vi "Graphics-Get Plot Properties.vi"(0 "Plot in":refnum<vi>, 11 "error in (no error)":errorcluster) -> (4 "Plot out":refnum<vi>, 8 "properties":T1, 15 "error out":errorcluster)   [LabVIEW 2020]
uses:
  Graphics-Plot Properties.ctl
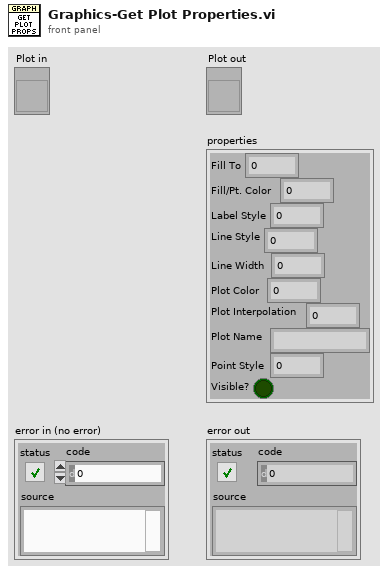
[diagram p1: front panel]
types:
  T1 = typedef "Graphics-Plot Properties.ctl" = cluster{"Fill To":i16, "Fill/Pt. Color":u32, "Label Style":u8, "Line Style":u8, "Line Width":u8, "Plot Color":u32, "Plot Interpolation":u8, "Plot Name":string, "Point Style":u8, "Visible?":bool}
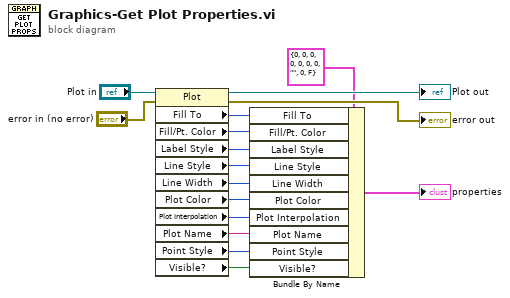
[diagram p0: block diagram]
diagram:
  n1 = property class="Plot"(reference="Plot in", error in="error in (no error)") -> (reference out=→"Plot out":refnum<vi>, error out=→"error out":errorcluster, "Fill To"=w11:i16, "Fill/Pt. Color"=w10:u32, "Label Style"=w9:u8, "Line Style"=w8:u8, "Line Width"=w7:u8, "Plot Color"=w6:u32, "Plot Interpolation"=w5:u8, "Plot Name"=w4:string, "Point Style"=w3:u8, "Visible?"=w2:bool)
  n2 = Bundle By Name(cluster=T1 {"Fill To"=0, "Fill/Pt. Color"=0, "Label Style"=0, "Line Style"=0, "Line Width"=0, "Plot Color"=0, "Plot Interpolation"=0, "Plot Name"="", "Point Style"=0, "Visible?"=FALSE} ("plot properties"), "Fill To"=w11, "Fill/Pt. Color"=w10, "Label Style"=w9, "Line Style"=w8, "Line Width"=w7, "Plot Color"=w6, "Plot Interpolation"=w5, "Plot Name"=w4, "Point Style"=w3, "Visible?"=w2) -> (→"properties":T1)
